vi "Parse HTML for Images.vi"(5 "Parent Path\n(Empty Path)":path, 6 "Report Text":string) -> (1 "Image Paths":path[](array[path]), 2 "Report Text for MHTML":string)   [LabVIEW 2011]
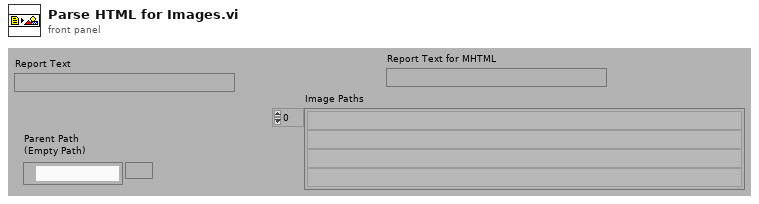
[diagram p1: front panel]
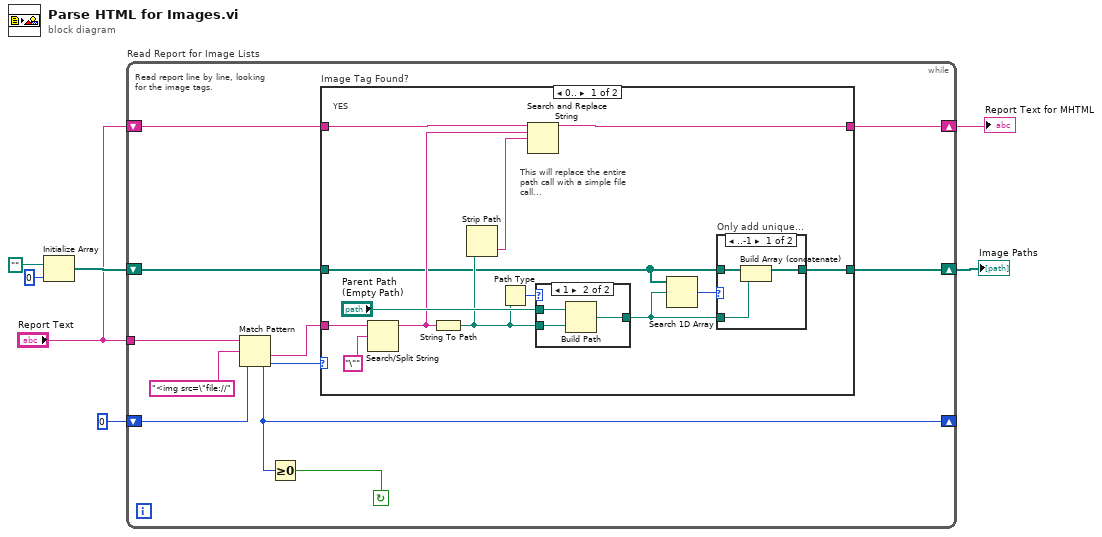
[diagram p0: block diagram]
diagram:
  n1 = Initialize Array(path "", 0 ("Dimension Size")) -> (w6:path[])
  n2 = while "Read Report for Image Lists" {
    shift-left: "Report Text" -> [w10]
    shift-right: [w9] -> w2
    tunnel: "Report Text" -> [w11]
    shift-left: 0 ("Dimension Size") -> [w13]
    shift-right: [w12] -> _
    shift-left: w6 -> [w15]
    shift-right: [w14] -> w7
    stop <- w8 continue-if-true
    # "Read report line by line, looking\nfor the image tags."
    n3 = Match Pattern(string=w11, regular expression="<img src=\"file://", offset (0)=w13) -> (after substring=w16:string, offset past match=w12:i32)  [unwired: 2 out]
    n4 = Greater Or Equal To 0?(x=w12) -> (x >= 0?=w8:bool)
    n5 = case "Image Tag Found?" shown="0.." w12 {
      tunnel: w16 -> [w26 _]
      tunnel: [w30 w40] -> w14
      tunnel: w15 -> [w20 w40]
      tunnel: [w24 w39] -> w9
      tunnel: w10 -> [w25 w39]
      frame 0.. {
        # "This will replace the entire\npath call with a simple file\ncall..."
        # "YES"
        n6 = Search/Split String(string=w26, search string/char (-)="\"") -> (substring before match=w22:string)  [unwired: 3 out]
        n7 = String To Path(string=w22) -> (path=w23:path)
        n8 = Strip Path(path=w23) -> (name=w21:string)  [unwired: 1 out]
        n9 = Path Type(1:w23) -> (0:w27:i16)
        n10 = Search and Replace String(input string=w25, search string=w22, replace string=w21) -> (result string=w24:string)  [unwired: 1 in, 7 out]
        n11 = case shown="1" w27 {
          tunnel: [w35 w38] -> w19
          tunnel: w23 -> [w35 w37]
          tunnel: "Parent Path\n(Empty Path)" -> [_ w36]
          frame 0, Default {
          }
          frame 1 {
            n12 = Build Path(base path=w36, name or relative path=w37) -> (appended path=w38:path)
          }
        }
        n13 = Search 1D Array(1D array=w20, element=w19) -> (index of element=w18:i32)  [unwired: 1 out]
        n14 = case "Only add unique..." shown="..-1" w18 {
          tunnel: [w33 w34] -> w30
          tunnel: w20 -> [w32 w34]
          tunnel: w19 -> [w31 _]
          frame ..-1 {
            n15 = Build Array (concatenate)(w32, w31) -> (w33:path[])
          }
          frame 0.. {
          }
        }
      }
      frame -1, Default {
        # "NO"
      }
    }
  }
  "Image Paths" <- w7
  "Report Text for MHTML" <- w2
